vi "stm_GetIDfromName.vi"(9 "Name":string, 11 "MetaData":T2[](array[typedef])) -> (1 "Found":bool, 3 "Meta ID":T1)   [LabVIEW 2010]
doc: "This VI looks up the Meta data index using the Meta data name.\n\nCopyright 2015, 2016, 2017 National Instruments Corporation\n\nLicensed under the Apache License, Version 2.0 (the \"License\"); you may not use this file except in compliance with the License.\n\n You may obtain a copy of the License at\n\n http://www.apache.org/licenses/LICENSE-2.0\n\nUnless required by applicable law or agreed to in writing, software distributed under the License is distributed on an \"AS IS\" BASIS, WITHOUT WARRANTIES OR CONDITIONS OF ANY KIND, either express or implied.\n\nSee the License for the specific language governing permissions and limitations under the License."
uses:
  stm_MetaElement.ctl
  stm_MetaID.ctl
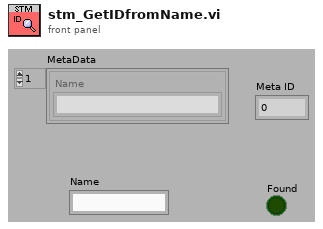
[diagram p1: front panel]
types:
  T1 = typedef "stm_MetaID.ctl" = u16
  T2 = typedef "stm_MetaElement.ctl" = cluster{"Name":string}
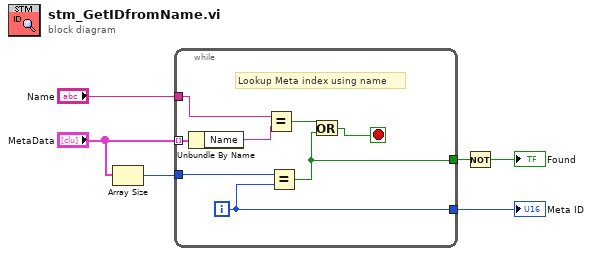
[diagram p0: block diagram]
diagram:
  n1 = Array Size(array="MetaData") -> (size(s)=w5:i32)
  n2 = while {
    tunnel: "MetaData" -> [w8] mode=indexing
    tunnel: w5 -> [w11]
    tunnel: "Name" -> [w14]
    tunnel: [w10] -> w3
    tunnel: [w9] -> w2
    i -> [w10]
    stop <- w12 stop-if-true
    # "Lookup Meta index using name"
    n3 = Unbundle By Name(w8) -> ("Name"=w7:string)
    n4 = Equal?(x=w14, y=w7) -> (x = y?=w13:bool)
    n5 = Equal?(x=w11, y=w10) -> (x = y?=w9:bool)
    n6 = Or(x=w13, y=w9) -> (x .or. y?=w12:bool)
  }
  "Meta ID" <- w3
  n7 = Not(x=w2) -> (.not. x?=→"Found":bool)
